vi "Write Room No.vi"(8 "error in (no error)":errorcluster, 10 "Room No":string, 11 "Room Service Base in":refnum<class "Room Service Base.lvclass">) -> (0 "error out":errorcluster, 3 "Room Service Base out":refnum<class "Room Service Base.lvclass">)   [LabVIEW 2023, in "Room Service Types.lvlib" / "Room Service Base.lvclass"]
uses:
  Room Service Base.lvclass
  Room Service Base.lvclass/Room Service Base.ctl
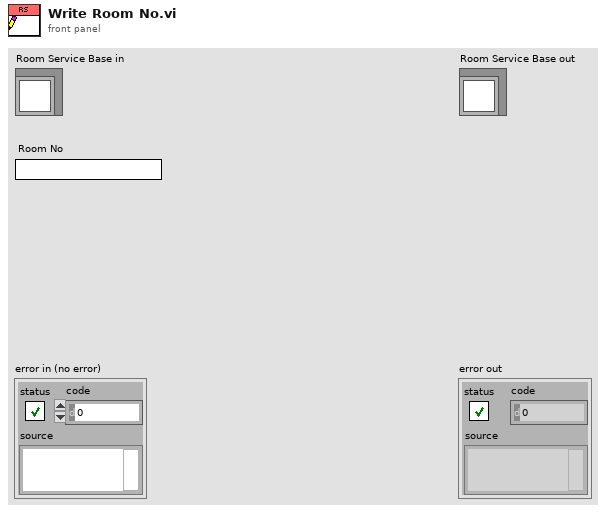
[diagram p1: front panel]
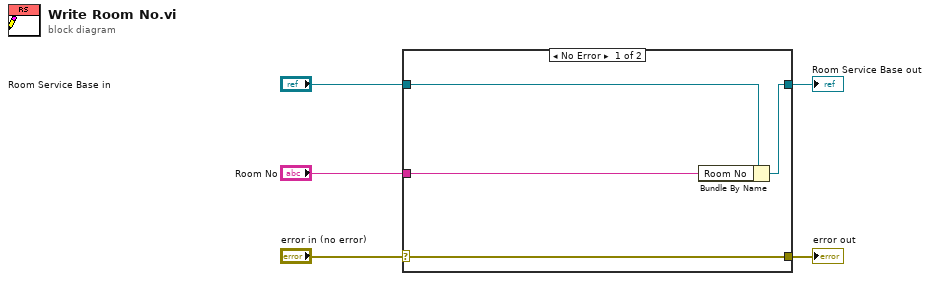
[diagram p0: block diagram]
diagram:
  n1 = case shown="No Error" "error in (no error)" {
    selector: "error in (no error)" -> [w9 w10]
    tunnel: [w9 w10] -> w4
    tunnel: [w7 w11] -> w2
    tunnel: "Room Service Base in" -> [w8 w11]
    tunnel: "Room No" -> [w6 _]
    frame No Error {
      n2 = Bundle By Name(cluster=w8, "Room No"=w6) -> (w7:refnum<class "Room Service Base.lvclass">)
    }
    frame Error {
    }
  }
  "error out" <- w4
  "Room Service Base out" <- w2
